vi "Set Visible Messages.vi"(8 "error in (no error)":errorcluster, 10 "Messages":set{string}(c389), 11 "Chronological List in":refnum<class "Chronological List.lvclass">) -> (0 "error out":errorcluster, 3 "Chronological List out":refnum<class "Chronological List.lvclass">)   [LabVIEW 2020, in "Chronological List.lvclass"]
uses:
  Chronological List.lvclass
  Chronological List.lvclass/Chronological List.ctl
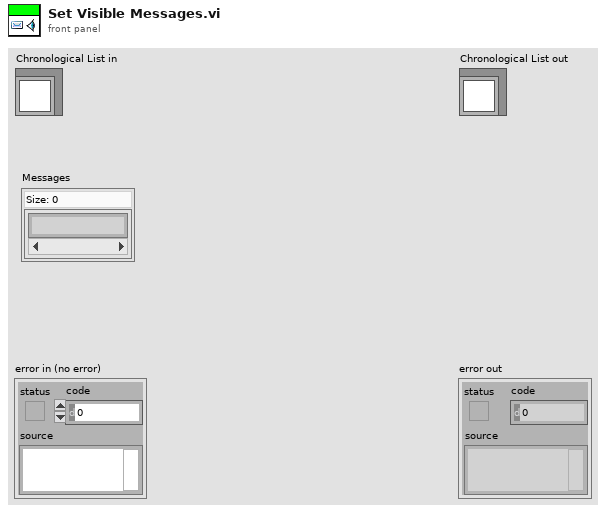
[diagram p1: front panel]
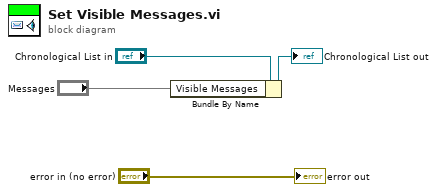
[diagram p0: block diagram]
diagram:
  n1 = Bundle By Name(cluster="Chronological List in", "Visible Messages"="Messages") -> (→"Chronological List out":refnum<class "Chronological List.lvclass">)
  "error out" <- "error in (no error)"
